vi "Close.vi"(8 "error in (no error)":errorcluster, 11 "FPGA:R-Series in":refnum<class "R-Series.lvclass">) -> (0 "error out":errorcluster, 3 "FPGA:R-Series out":refnum<class "R-Series.lvclass">)   [LabVIEW 2025, in "FPGA.lvlib" / "R-Series.lvclass"]
uses:
  R-Series.lvclass
  R-Series.lvclass/R-Series.ctl
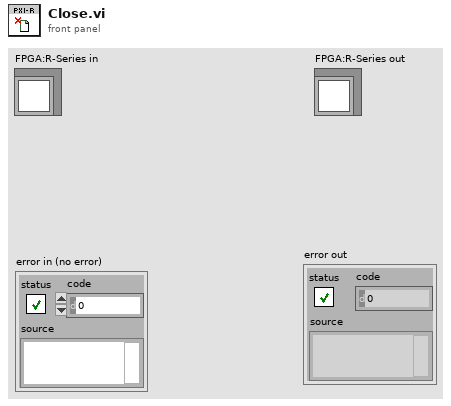
[diagram p1: front panel]
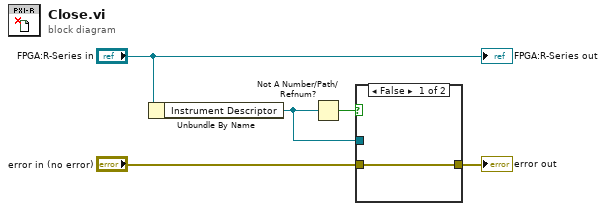
[diagram p0: block diagram]
diagram:
  n1 = Unbundle By Name("FPGA:R-Series in") -> ("Instrument Descriptor"=w1:refnum<k15>)
  n2 = Not A Number/Path/Refnum?(number/path/refnum=w1) -> (NaN/Path/Refnum?=w2:bool)
  n3 = case shown="False" w2 {
    tunnel: "error in (no error)" -> [w6 w7]
    tunnel: [w6 w7] -> w3
    tunnel: w1 -> [_ _]
    frame False {
    }
    frame True {
    }
  }
  "error out" <- w3
  "FPGA:R-Series out" <- "FPGA:R-Series in"
